vi "libssh2_session_disconnect_ex.vi"(7 "lang":string, 8 "error in (no error)":errorcluster, 9 "description":string, 10 "reason":i32, 11 "session":T1) -> (0 "error out":errorcluster)   [LabVIEW 2017, in "libssh2.lvlib"]
doc: "Disconnect a session with a custom reason and language tag."
uses:
  libssh2.lvlib
  Session Refnum.ctl
  Not A Session.vi
  <vilib>/Utility/error.llb/Error Cluster From Error Code.vi
  Global Settings.vi
  Read Session Refnum.vi
  <vilib>/Utility/semaphor.llb/Acquire Semaphore.vi
  <vilib>/Utility/semaphor.llb/Release Semaphore.vi
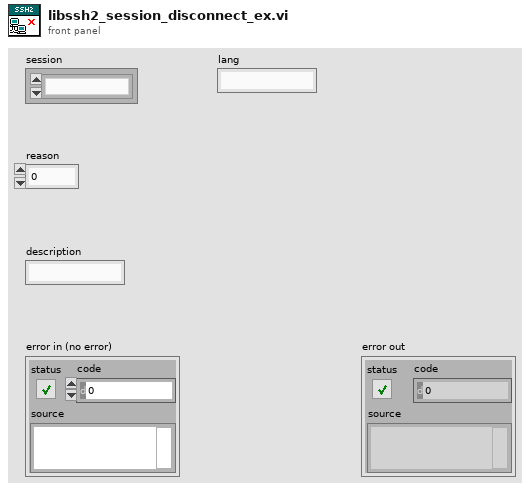
[diagram p1: front panel]
types:
  T1 = typedef "libssh2.lvlib/Session Refnum.ctl" = refnum<k1>
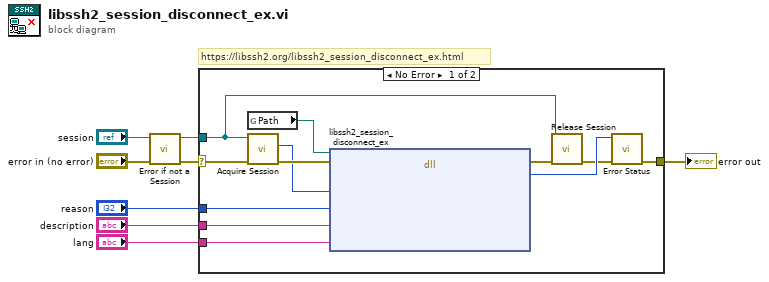
[diagram p0: block diagram]
diagram:
  # "https://libssh2.org/libssh2_session_disconnect_ex.html"
  n1 = call "Error if not a Session.vi"("error in (no error)"="error in (no error)", "session"="session") -> ("error out"=w3:errorcluster, "session out"=w1:T1)  [unwired: 8 in]
  n2 = case shown="No Error" w3 {
    selector: w3 -> [w17 w21]
    tunnel: [w16 w21] -> w8
    tunnel: "reason" -> [w20 _]
    tunnel: "description" -> [w19 _]
    tunnel: "lang" -> [w18 _]
    tunnel: w1 -> [w9 _]
    frame No Error {
      n3 = global read "Global Settings.vi" "Path"() -> (w12:path)
      n4 = call "Acquire Session.vi"("error in (no error)"=w17, "session"=w9) -> ("error out"=w14:errorcluster, "LIBSSH2_SESSION*"=w13:u64)  [unwired: 7 in, 1 out]
      n5 = dll-call lib="?" fn="libssh2_session_disconnect_ex"(path in=w12, error in=w14, "session"=w13, "reason"=w20, "description"=w19, "lang"=w18) -> (error out=w15:errorcluster, "return value"=w11:i32)  [unwired: 5 in, 1 out]
      n6 = call "Release Session.vi"("error in (no error)"=w15, "session"=w9) -> ("error out"=w10:errorcluster)  [unwired: 9 in]
      n7 = call "Error Status.vi"("error in (no error)"=w10, "return value"=w11) -> ("error out"=w16:errorcluster)  [unwired: 8 in, 1 out]
    }
    frame Error {
    }
  }
  "error out" <- w8
